vi "Getting Started with Order Analysis.vi"() -> ()   [LabVIEW 2017]
doc: "This VI demonstrates each of the order analysis features. This VI includes the following functions:\n1. Waveform and Speed Profile\n2. Colormap\n3. Order Spectrum\n4. Order Magnitude and Phase\n5. Waterfall Plot\n6. Cascade Plot\n7. Orbit Plot\n8. Timebase Plot\n9. Polar Plot\n10. Shaft Centerline Plot"
panel:
  in  "STOP":bool
  out "left_top":bool
  out "status":string
  out "selected item":string
  in  "tree":string(tree)="Toolkit Features"
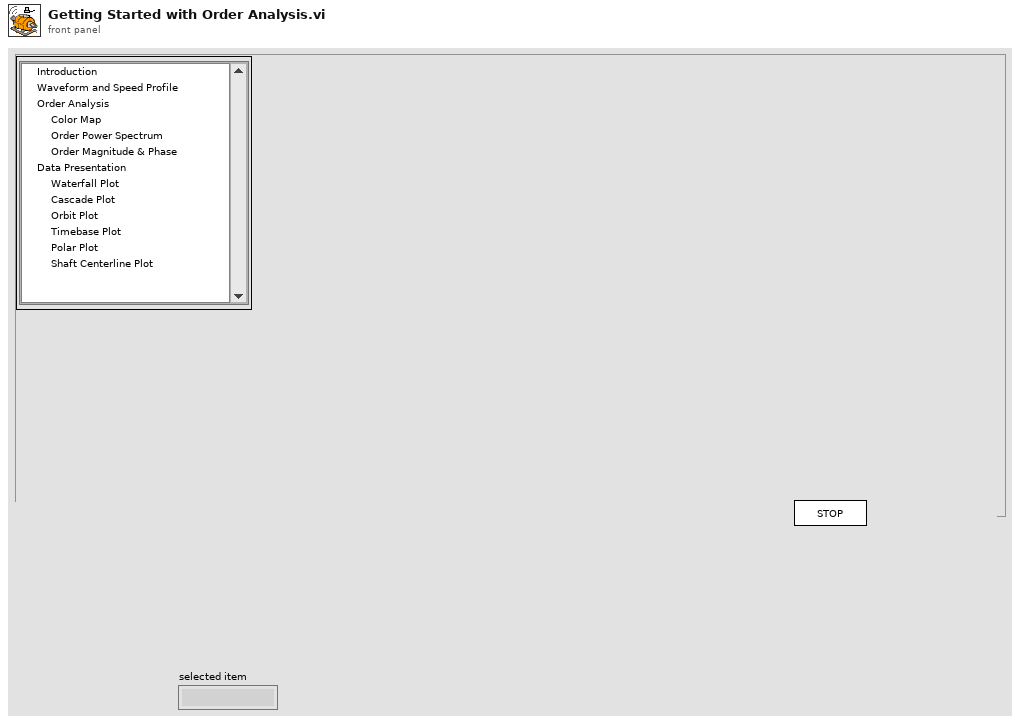
[diagram p1: front panel]
types:
  T1 = typedef "LVPositionTypeDef.ctl" = cluster{"Left":i32, "Top":i32}
  T2 = enum32{"Bad", "Idle", "Run top level", "Running"}
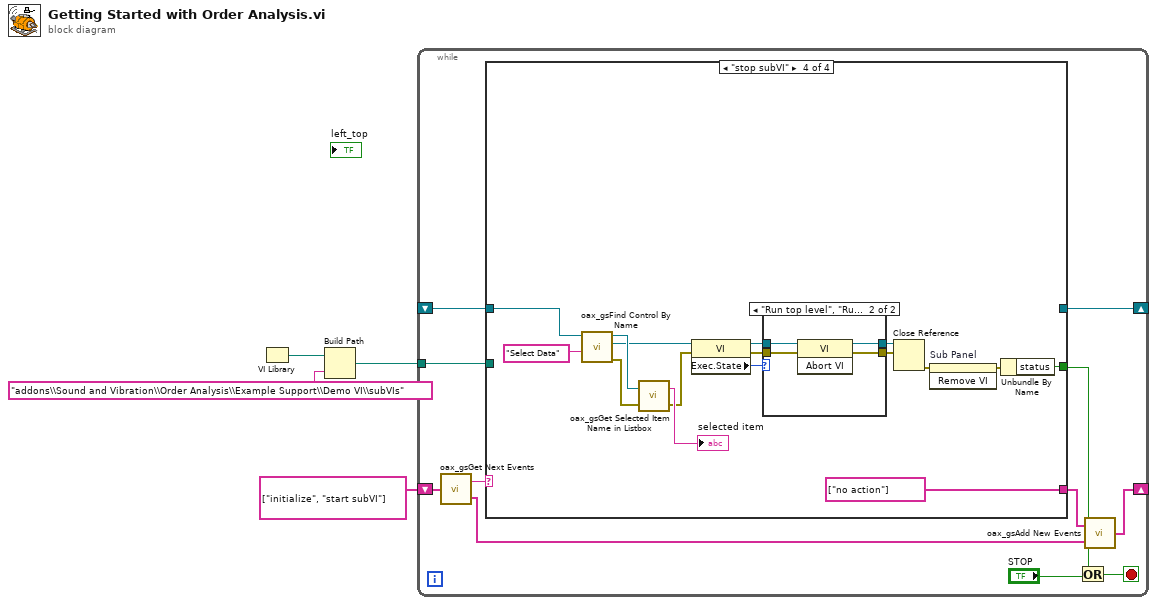
[diagram p0: block diagram]
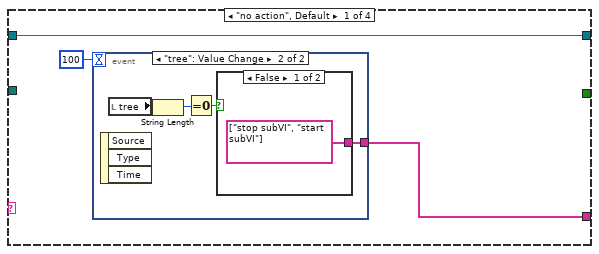
[diagram p2: hidden frame]
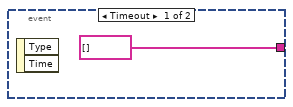
[diagram p3: hidden frame]
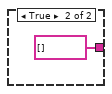
[diagram p4: hidden frame]
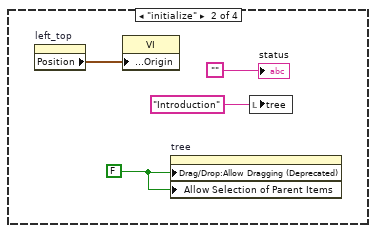
[diagram p5: hidden frame]
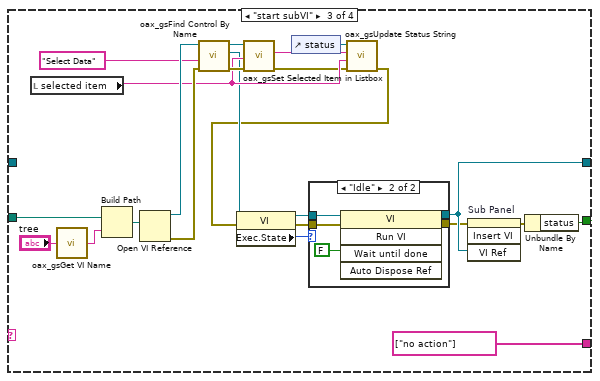
[diagram p6: hidden frame]
diagram:
  n1 = VI Library() -> (path=w2:path)
  n2 = Build Path(base path=w2, name or relative path="addons\\Sound and Vibration\\Order Analysis\\Example Support\\Demo VI\\subVIs") -> (appended path=w1:path)
  n3 = while {
    tunnel: w1 -> [w15]
    shift-right: [w14] -> _
    shift-left: _ -> [w13]
    shift-right: [w8] -> _
    shift-left: string[] ["initialize", "start subVI"] -> [w12]
    stop <- w5 stop-if-true
    n4 = call <vilib>:"oax_gsGet Next Events.vi"("event queue in"=w12) -> ("next event"=w11:string, "event queue out"=w10:string[])
    n5 = case shown="\"stop subVI\"" w11 {
      tunnel: w15 -> [_ _ w52 _]
      tunnel: [w18 _ w50 _] -> w14
      tunnel: w13 -> [w18 _ _ w71]
      tunnel: [_ _ w51 w75] -> w6
      tunnel: [w16 _ string[] ["no action"] string[] ["no action"]] -> w9
      frame "no action", Default {
        n6 = event shown="[1] \"tree\": Value Change" {
          selector: _ -> [_ _]
          dyn-events: _ -> [_ _]
          timeout: 100 -> [_ _]
          tunnel: [string[] [] ("f") w23] -> w16
          event Timeout {
            n7 = event-data() -> ()  [unwired: 1 in, 2 out]
          }
          event "tree": Value Change {
            n8 = event-data() -> ()  [unwired: 1 in, 3 out]
            n9 = local read "tree"() -> (w21:string)
            n10 = String Length(string=w21) -> (length=w22:i32)
            n11 = Equal To 0?(x=w22) -> (x = 0?=w20:bool)
            n12 = case shown="False" w20 {
              tunnel: [string[] ["stop subVI", "start subVI"] string[] []] -> w23
              frame False {
              }
              frame True {
              }
            }
          }
        }
      }
      frame "initialize" {
        w27 = FALSE ("Allow Dragging")
        n13 = property on="left_top" class="Bool (strict)"() -> ("Position"=w26:T1)  [unwired: 2 in, 2 out]
        n14 = property class="VI"("Front Panel Window:Origin"=w26) -> ()  [unwired: 2 in, 2 out]
        n15 = property on="tree" class="Tree (strict)"("Drag/Drop:Allow Dragging (Deprecated)"=w27, "Allow Selection of Parent Items"=w27) -> ()  [unwired: 2 in, 2 out]
        n16 = local write "tree"("Introduction" ("tree")) -> ()
        "status" <- ""
      }
      frame "start subVI" {
        n17 = local read "selected item"() -> (w37:string)
        n18 = call <vilib>:"oax_gsGet VI Name.vi"("tree"="tree") -> ("vi name"=w47:string)
        n19 = Build Path(base path=w52, name or relative path=w47) -> (appended path=w46:path)
        n20 = Open VI Reference(vi path=w46) -> (vi reference=w42:refnum<vi>, error out=w43:errorcluster)  [unwired: 5 in]
        n21 = call <vilib>:"oax_gsFind Control By Name.vi"("error in (no error)"=w43, "control name"="Select Data", "vi refnum in"=w42) -> ("error out"=w39:errorcluster, "vi refnum out"=w34:refnum<vi>, "control refnum"=w40:refnum<vi>)  [unwired: 6 in]
        n22 = call <vilib>:"oax_gsSet Selected Item in Listbox.vi"("error in (no error)"=w39, "item name"=w37, "control refnum"=w40) -> ("error out"=w35:errorcluster, "actual item name"=w36:string)  [unwired: 6 in, 1 out]
        n23 = control-ref of="status"() -> (w38:refnum<vi>)
        n24 = call <vilib>:"oax_gsUpdate Status String.vi"("error in (no error)"=w35, "old status"=w37, "new status"=w36, "Ctl Refnum"=w38) -> ("error out"=w33:errorcluster)  [unwired: 3 in]
        n25 = property class="VI"(reference=w34, error in=w33) -> (reference out=w31:refnum<vi>, error out=w32:errorcluster, "Exec.State"=w30:T2)
        n26 = case shown="\"Idle\"" w30 {
          tunnel: [w54 w59] -> w50
          tunnel: [w53 w57] -> w45
          tunnel: w32 -> [w53 w56]
          tunnel: w31 -> [w54 w55]
          frame "Bad", Default {
          }
          frame "Idle" {
            n27 = invoke class="VI" method="Run VI"(reference=w55, error in=w56, "Wait until done"=FALSE) -> (reference out=w59:refnum<vi>, error out=w57:errorcluster)  [unwired: 2 in, 3 out]
          }
        }
        n28 = invoke on="Sub Panel" class="SubPanel" method="Insert VI"(error in=w45, "VI Ref"=w50) -> (error out=w44:errorcluster)  [unwired: 2 in, 3 out]
        n29 = Unbundle By Name(w44) -> ("status"=w51:bool)
      }
      frame "stop subVI" {
        n30 = call <vilib>:"oax_gsFind Control By Name.vi"("control name"="Select Data", "vi refnum in"=w71) -> ("error out"=w68:errorcluster, "vi refnum out"=w66:refnum<vi>, "control refnum"=w69:refnum<vi>)  [unwired: 7 in]
        n31 = call <vilib>:"oax_gsGet Selected Item Name in Listbox.vi"("error in (no error)"=w68, "ctrl reference"=w69) -> ("error out"=w65:errorcluster, "selected item"=→"selected item":string)
        n32 = property class="VI"(reference=w66, error in=w65) -> (reference out=w62:refnum<vi>, error out=w61:errorcluster, "Exec.State"=w64:T2)
        n33 = case shown="\"Run top level\", \"Running\"" w64 {
          tunnel: [w77 w79] -> w63
          tunnel: w62 -> [w77 w80]
          tunnel: w61 -> [w76 w81]
          tunnel: [w76 w78] -> w60
          frame "Bad", Default {
          }
          frame "Run top level", "Running" {
            n34 = invoke class="VI" method="Abort VI"(reference=w80, error in=w81) -> (reference out=w79:refnum<vi>, error out=w78:errorcluster)  [unwired: 1 in, 1 out]
          }
        }
        n35 = Close Reference(reference=w63, error in (no error)=w60) -> (error out=w73:errorcluster)
        n36 = invoke on="Sub Panel" class="SubPanel" method="Remove VI"(error in=w73) -> (error out=w72:errorcluster)  [unwired: 2 in, 2 out]
        n37 = Unbundle By Name(w72) -> ("status"=w75:bool)
      }
    }
    n38 = Or(x=w6, y="STOP") -> (x .or. y?=w5:bool)
    n39 = call <vilib>:"oax_gsAdd New Events.vi"("event in"=w10, "new events"=w9) -> ("event out"=w8:string[])
  }
